vi "‚liminer rectangle2‚crans.vi"(0 "Chaine d'entrée":string, 7 "entrée d'erreur (pas d'erreur)":errorcluster) -> (16 "taille (S1)":u32, 17 "taille (S3)":u32, 18 "taille (S2)":u32, 19 "taille (S4)":u32, 20 "S1":cluster{"X (S2;b1) ":u32, "Y (S2;b1)":u32}, 22 "S2":cluster{"X (S2;b1) ":u32, "Y (S2;b1)":u32}, 24 "S3":cluster{"X (S2;b1) ":u32, "Y (S2;b1)":u32}, 26 "S4":cluster{"X (S2;b1) ":u32, "Y (S2;b1)":u32}, 27 "sortie d'erreur":errorcluster)   [LabVIEW 2013]
uses:
  <vilib>/regexp/Match Regular Expression.xnode
panel:
  out "X1":u32
  out "Y1":u32
  out "Chaine (Signature 1; block 4)":string
  out "Chaine (Signature 1; block 3)":string
  out "Chaine (Signature 2)":string
  out "Chaine (Signature 1)":string
  out "X3":u32
  out "Y3":u32
  out "X2":u32
  out "Y2":u32
  out "X4":u32
  out "Y4":u32
  # "Caméra 1"
  # "Ce sous-vi permet de convertir les informations \nrecu pour chaque signature en une information \nde position (coordonnées x et y) et une \ninformation de taille"
  # "Caméra 2"
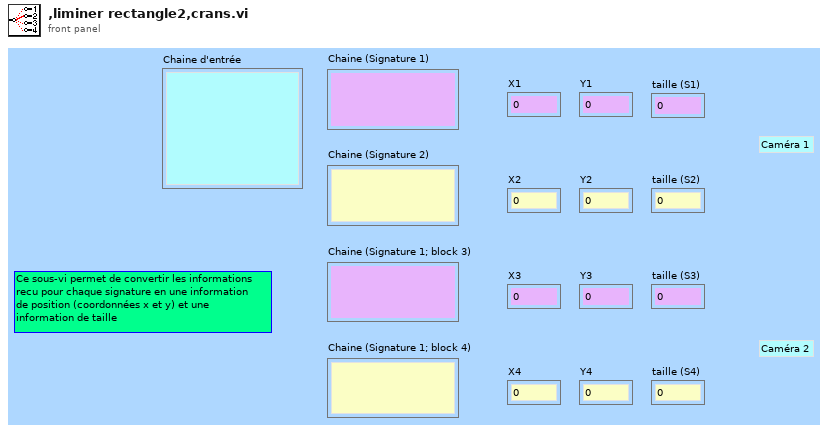
[diagram p1: front panel]
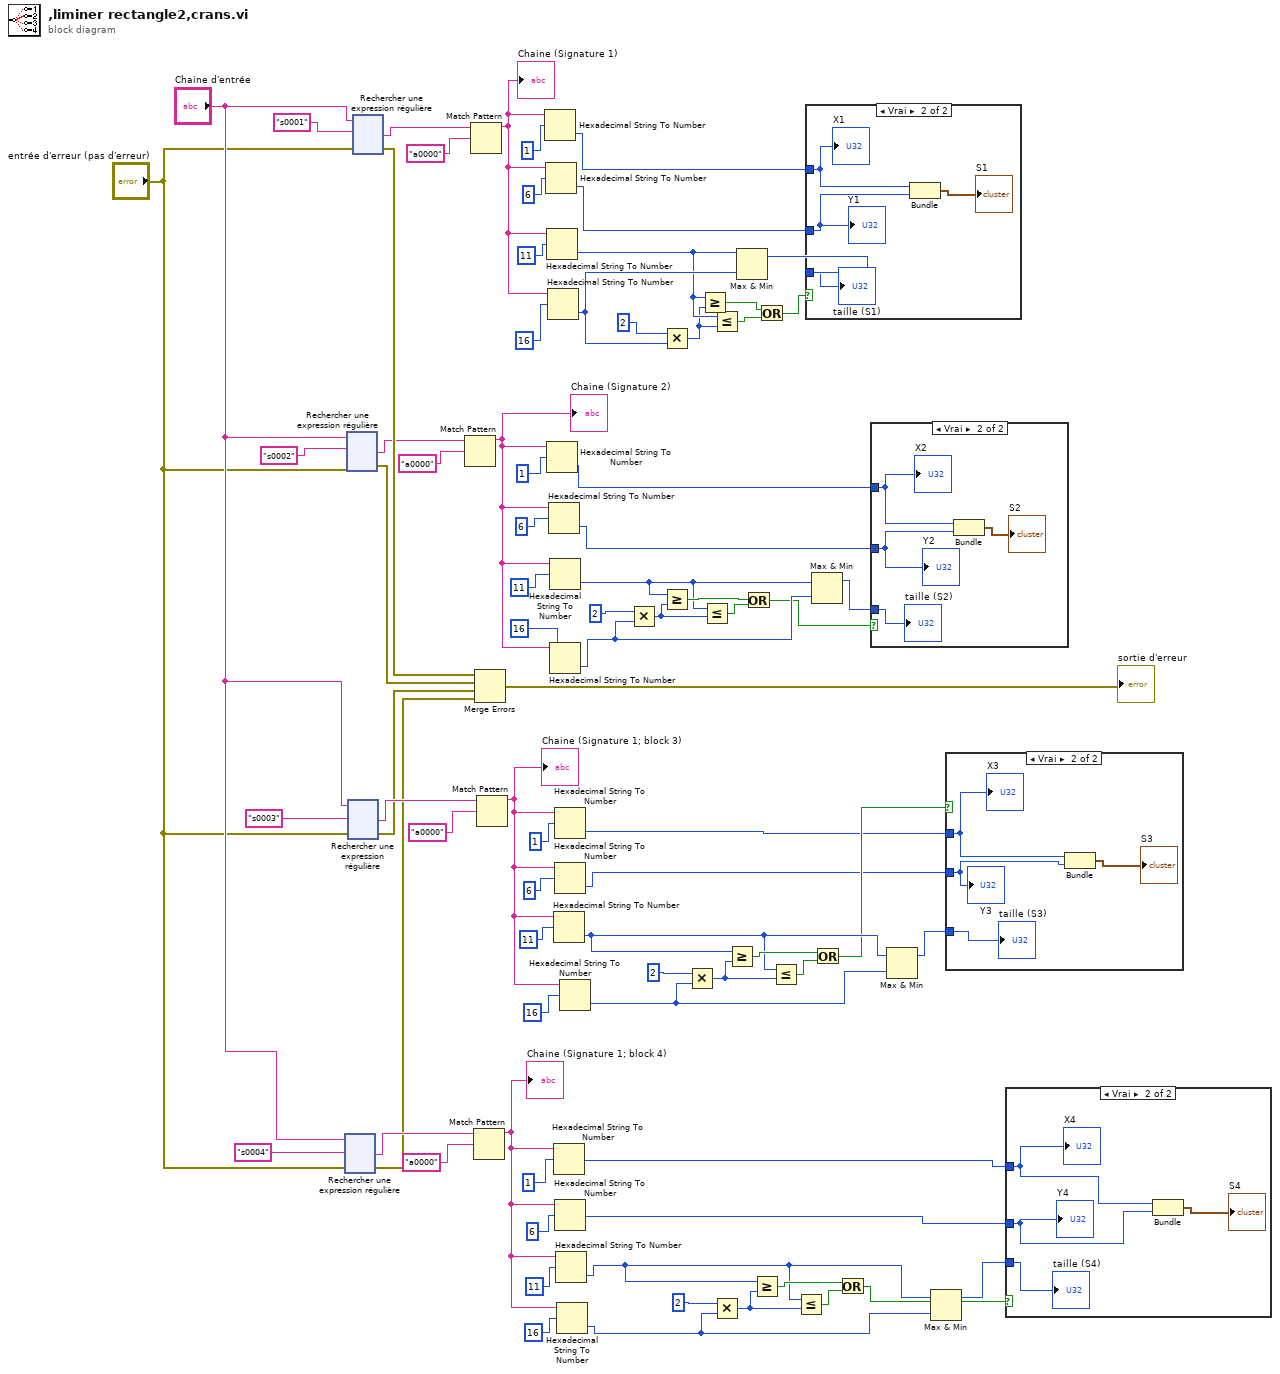
[diagram p0: block diagram]
diagram:
  n1 = xnode "Rechercher une expression régulière"("chaîne en entrée"="Chaine d'entrée", "expression régulière"="s0004", "entrée d'erreur"="entrée d'erreur (pas d'erreur)") -> ("après la correspondance"=w46:string, "sortie d'erreur"=w43:errorcluster)  [unwired: 3 in, 3 out]
  n2 = xnode "Rechercher une expression régulière"("chaîne en entrée"="Chaine d'entrée", "expression régulière"="s0002", "entrée d'erreur"="entrée d'erreur (pas d'erreur)") -> ("après la correspondance"=w60:string, "sortie d'erreur"=w45:errorcluster)  [unwired: 3 in, 3 out]
  n3 = xnode "Rechercher une expression régulière"("chaîne en entrée"="Chaine d'entrée", "expression régulière"="s0003", "entrée d'erreur"="entrée d'erreur (pas d'erreur)") -> ("après la correspondance"=w53:string, "sortie d'erreur"=w44:errorcluster)  [unwired: 3 in, 3 out]
  n4 = xnode "Rechercher une expression régulière"("chaîne en entrée"="Chaine d'entrée", "expression régulière"="s0001", "entrée d'erreur"="entrée d'erreur (pas d'erreur)") -> ("après la correspondance"=w70:string, "sortie d'erreur"=w74:errorcluster)  [unwired: 3 in, 3 out]
  n5 = Match Pattern(string=w60, regular expression="a0000") -> (before substring=w61:string)  [unwired: 1 in, 3 out]
  "Chaine (Signature 2)" <- w61
  n6 = Match Pattern(string=w70, regular expression="a0000") -> (before substring=w67:string)  [unwired: 1 in, 3 out]
  "Chaine (Signature 1)" <- w67
  n7 = Match Pattern(string=w46, regular expression="a0000") -> (before substring=w47:string)  [unwired: 1 in, 3 out]
  "Chaine (Signature 1; block 4)" <- w47
  n8 = Merge Errors(w74, w45, w44, w43) -> (→"sortie d'erreur":errorcluster)
  n9 = Match Pattern(string=w53, regular expression="a0000") -> (before substring=w54:string)  [unwired: 1 in, 3 out]
  "Chaine (Signature 1; block 3)" <- w54
  n10 = Hexadecimal String To Number(string=w67, offset=1) -> (number=w33:u32)  [unwired: 1 in, 1 out]
  n11 = Hexadecimal String To Number(string=w67, offset=6) -> (number=w34:u32)  [unwired: 1 in, 1 out]
  n12 = Hexadecimal String To Number(string=w67, offset=11) -> (number=w23:u32)  [unwired: 1 in, 1 out]
  n13 = Hexadecimal String To Number(string=w61, offset=1) -> (number=w32:u32)  [unwired: 1 in, 1 out]
  n14 = Hexadecimal String To Number(string=w67, offset=16) -> (number=w39:u32)  [unwired: 1 in, 1 out]
  n15 = Hexadecimal String To Number(string=w61, offset=6) -> (number=w29:u32)  [unwired: 1 in, 1 out]
  n16 = Hexadecimal String To Number(string=w61, offset=11) -> (number=w27:u32)  [unwired: 1 in, 1 out]
  n17 = Hexadecimal String To Number(string=w61, offset=16) -> (number=w37:u32)  [unwired: 1 in, 1 out]
  n18 = Hexadecimal String To Number(string=w54, offset=11) -> (number=w15:u32)  [unwired: 1 in, 1 out]
  n19 = Hexadecimal String To Number(string=w47, offset=1) -> (number=w4:u32)  [unwired: 1 in, 1 out]
  n20 = Hexadecimal String To Number(string=w54, offset=1) -> (number=w13:u32)  [unwired: 1 in, 1 out]
  n21 = Hexadecimal String To Number(string=w54, offset=6) -> (number=w12:u32)  [unwired: 1 in, 1 out]
  n22 = Hexadecimal String To Number(string=w47, offset=6) -> (number=w1:u32)  [unwired: 1 in, 1 out]
  n23 = Hexadecimal String To Number(string=w47, offset=11) -> (number=w6:u32)  [unwired: 1 in, 1 out]
  n24 = Hexadecimal String To Number(string=w47, offset=16) -> (number=w5:u32)  [unwired: 1 in, 1 out]
  n25 = Hexadecimal String To Number(string=w54, offset=16) -> (number=w16:u32)  [unwired: 1 in, 1 out]
  n26 = Multiply(x=2, y=w37) -> (x*y=w26:u32)
  n27 = Multiply(x=2, y=w39) -> (x*y=w22:u32)
  n28 = Greater Or Equal?(x=w27, y=w26) -> (x >= y?=w28:bool)
  n29 = Multiply(x=2, y=w16) -> (x*y=w18:u32)
  n30 = Greater Or Equal?(x=w23, y=w22) -> (x >= y?=w24:bool)
  n31 = Less Or Equal?(x=w27, y=w26) -> (x <= y?=w25:bool)
  n32 = Less Or Equal?(x=w23, y=w22) -> (x <= y?=w21:bool)
  n33 = Multiply(x=2, y=w5) -> (x*y=w8:u32)
  n34 = Greater Or Equal?(x=w15, y=w18) -> (x >= y?=w19:bool)
  n35 = Max & Min(x=w23, y=w39) -> (max(x,y)=w35:u32)  [unwired: 1 out]
  n36 = Or(x=w28, y=w25) -> (x .or. y?=w31:bool)
  n37 = Greater Or Equal?(x=w6, y=w8) -> (x >= y?=w9:bool)
  n38 = Or(x=w24, y=w21) -> (x .or. y?=w36:bool)
  n39 = Less Or Equal?(x=w15, y=w18) -> (x <= y?=w17:bool)
  n40 = Less Or Equal?(x=w6, y=w8) -> (x <= y?=w7:bool)
  n41 = case shown="Vrai" w36 {
    tunnel: w35 -> [_ w80]
    tunnel: w34 -> [_ w81]
    tunnel: w33 -> [_ w82]
    frame False {
    }
    frame True {
      n42 = Bundle(w82, w81) -> (→"S1":cluster{u32, u32})  [unwired: 1 in]
      "Y1" <- w81
      "X1" <- w82
      "taille (S1)" <- w80
    }
  }
  n43 = Max & Min(x=w27, y=w37) -> (max(x,y)=w30:u32)  [unwired: 1 out]
  n44 = Or(x=w19, y=w17) -> (x .or. y?=w14:bool)
  n45 = Or(x=w9, y=w7) -> (x .or. y?=w3:bool)
  n46 = case shown="Vrai" w31 {
    tunnel: w32 -> [_ w86]
    tunnel: w30 -> [_ w84]
    tunnel: w29 -> [_ w85]
    frame False {
    }
    frame True {
      n47 = Bundle(w86, w85) -> (→"S2":cluster{u32, u32})  [unwired: 1 in]
      "Y2" <- w85
      "X2" <- w86
      "taille (S2)" <- w84
    }
  }
  n48 = Max & Min(x=w15, y=w16) -> (max(x,y)=w11:u32)  [unwired: 1 out]
  n49 = Max & Min(x=w6, y=w5) -> (max(x,y)=w2:u32)  [unwired: 1 out]
  n50 = case shown="Vrai" w14 {
    tunnel: w13 -> [_ w90]
    tunnel: w12 -> [_ w89]
    tunnel: w11 -> [_ w88]
    frame False {
    }
    frame True {
      n51 = Bundle(w90, w89) -> (→"S3":cluster{u32, u32})  [unwired: 1 in]
      "Y3" <- w89
      "X3" <- w90
      "taille (S3)" <- w88
    }
  }
  n52 = case shown="Vrai" w3 {
    tunnel: w4 -> [_ w94]
    tunnel: w2 -> [_ w92]
    tunnel: w1 -> [_ w93]
    frame False {
    }
    frame True {
      n53 = Bundle(w94, w93) -> (→"S4":cluster{u32, u32})  [unwired: 1 in]
      "Y4" <- w93
      "X4" <- w94
      "taille (S4)" <- w92
    }
  }
